vi "Read Camera By Name.vi"(8 "error in (no error)":errorcluster, 10 "Camera Name":string, 11 "Gantry Class in":refnum<class "Gantry Class.lvclass">) -> (0 "error out":errorcluster, 2 "Camera":T1, 3 "Gantry Class out":refnum<class "Gantry Class.lvclass">)   [LabVIEW 2011, in "Gantry Class.lvclass"]
uses:
  Gantry Class.lvclass
  Type Definitions/Gantry_Camera.ctl
  <vilib>/userdefined/High Color/IMAQdx.ctl
  Gantry Class.lvclass/Gantry Class.ctl
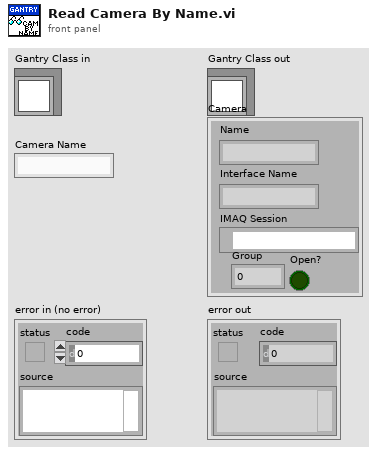
[diagram p1: front panel]
types:
  T1 = typedef "Gantry_Camera.ctl" = cluster{"Name":string, "IMAQ Session":T2, "Group":u32, "Open?":bool, "Interface Name":string}
  T2 = typedef "IMAQdx.ctl" = refnum<k21>
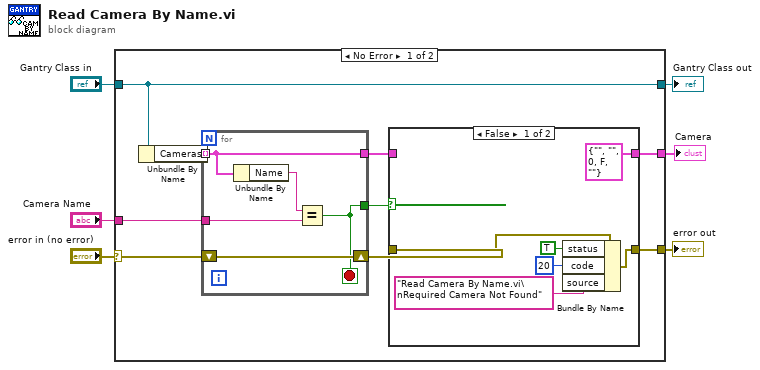
[diagram p0: block diagram]
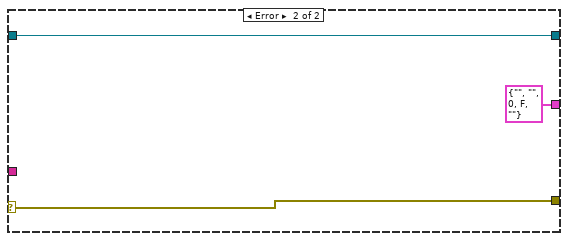
[diagram p3: hidden frame]
diagram:
  n1 = case shown="No Error" "error in (no error)" {
    selector: "error in (no error)" -> [w14 w30]
    tunnel: [w10 w30] -> w5
    tunnel: [w15 w31] -> w3
    tunnel: "Gantry Class in" -> [w15 w31]
    tunnel: [w7 T1 {"Name"="", "IMAQ Session"="", "Group"=0, "Open?"=FALSE, "Interface Name"=""} ("Camera")] -> w1
    tunnel: "Camera Name" -> [w12 _]
    frame No Error {
      n2 = Unbundle By Name(w15) -> ("Cameras"=w13:T1[])
      n3 = for {
        shift-right: [w25] -> w11
        shift-left: w14 -> [w25]
        tunnel: w13 -> [w26] mode=indexing
        tunnel: w12 -> [w27]
        tunnel: [w26] -> w8
        tunnel: [w24] -> w9
        stop <- w24 stop-if-true
        n4 = Unbundle By Name(w26) -> ("Name"=w28:string)
        n5 = Equal?(x=w28, y=w27) -> (x = y?=w24:bool)
      }
      n6 = case shown="False" w9 {
        tunnel: w11 -> [w21 w23]
        tunnel: [w20 w23] -> w10
        tunnel: w8 -> [_ w22]
        tunnel: [T1 {"Name"="", "IMAQ Session"="", "Group"=0, "Open?"=FALSE, "Interface Name"=""} ("Camera") w22] -> w7
        frame False {
          n7 = Bundle By Name(cluster=w21, "status"=TRUE, "code"=20, "source"="Read Camera By Name.vi\nRequired Camera Not Found") -> (w20:errorcluster)
        }
        frame True {
        }
      }
    }
    frame Error {
    }
  }
  "error out" <- w5
  "Gantry Class out" <- w3
  "Camera" <- w1
